vi "图像采集与保存-简单图像处理.vi"(9 "Grab":bool, 11 "Camera Name":refnum<k21>="cam0" caption="IMAQdx Session") -> ()   [LabVIEW 2022 SP3]
doc: "The Grab and Attributes Setup example VI allows the user to view the current attributes and settings, update attribute settings, acquire images continuously, and display the images in an image control."
uses:
  <vilib>/vision/driver/IMAQdx.llb/IMAQdx Acquisition Mode.ctl
  <vilib>/vision/driver/IMAQdx.llb/IMAQdx Buffer Number Mode.ctl
  <vilib>/vision/driver/NI_Vision_Acquisition_Software.lvlib
panel:
  out "Image out":T1(plugin-control)
  out "错误输出":errorcluster
  out "返回值":i32
  out "处理图片路径":path
  out "采集图片路径":path
  out "帧数":i32
  in  "采集帧间隔":i8
  in  "确定按钮":bool
  in  "Tab Control":T2(tab)
  in  "U32 Value Control":u32(slide) min=1 step=1 scale=1.0..4294967295.0
  in  "DBL Value Control":dbl(slide) min=2.2571161239684447 max=1000.0 step=1.0 scale=2.2571161239684447..1000.0
  in  "String Value Control":string
  in  "Enum Value Control":u32(ring) items=["Unicast", "Broadcast", "Multicast"]
  in  "Boolean Value Control":bool
  in  "Command Value Control":bool
  out "Tooltip":string="Gets/Sets the maximum number of outstanding events to queue."
  out "Units":string
  in  "Attribute Tree":string(tree)
  out "Frame Rate":dbl(knob) scale=0.0..100.0
  out "Image":T1(plugin-control)
  out "Buffer Number":u32
  in  "Stop":bool
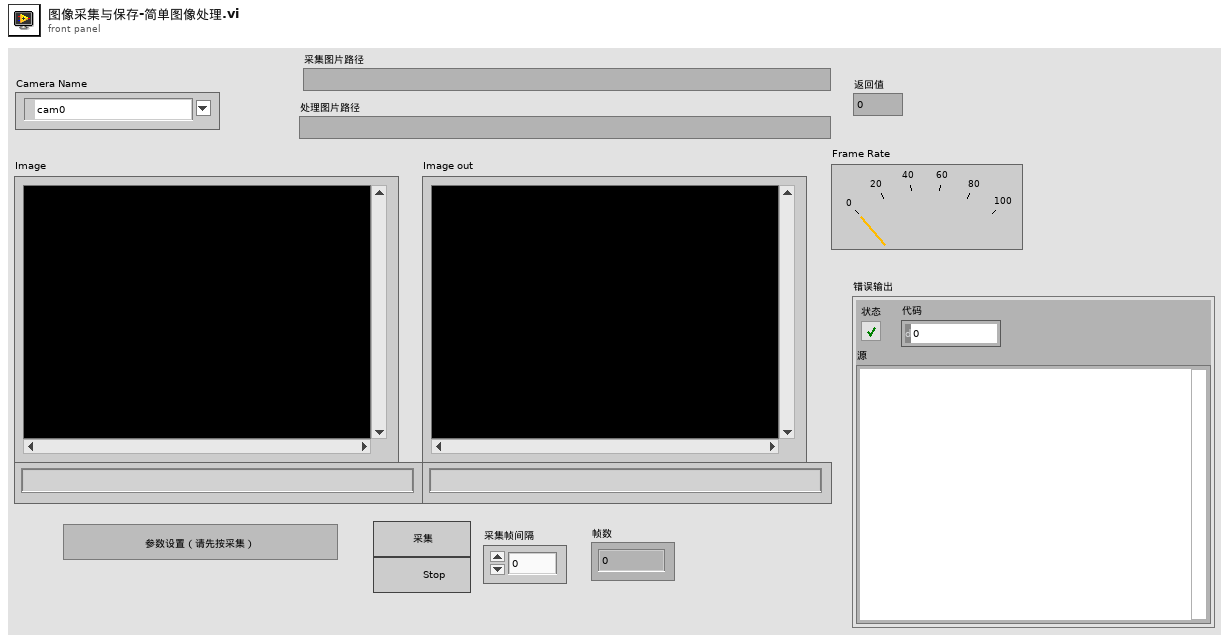
[diagram p1: front panel]
types:
  T1 = typedef "IMAQ Image.ctl" = refnum<image>
  T2 = enum32{"U32", "DBL", "String", "Enum", "Bool", "Command"}
  T3 = typedef "NI_Vision_Acquisition_Software.lvlib/IMAQdx Acquisition Mode.ctl" = enum32{"One Shot", "Continuous"}
  T4 = typedef "IMAQdx.ctl" = refnum<k21>
  T5 = cluster{"Tab Control":refnum<vi>, "U32 Value Control":refnum<vi>, "DBL Value Control":refnum<vi>, "String Value Control":refnum<vi>, "Enum Value Control":refnum<vi>, "Boolean Value Control":refnum<vi>, "Command Value Control":refnum<vi>}
  T6 = typedef "NI_Vision_Acquisition_Software.lvlib/IMAQdx Buffer Number Mode.ctl" = enum32{"Next", "Last", "Buffer Number", "Every", "Last New"}
  T7 = typedef "Image Type" = u32
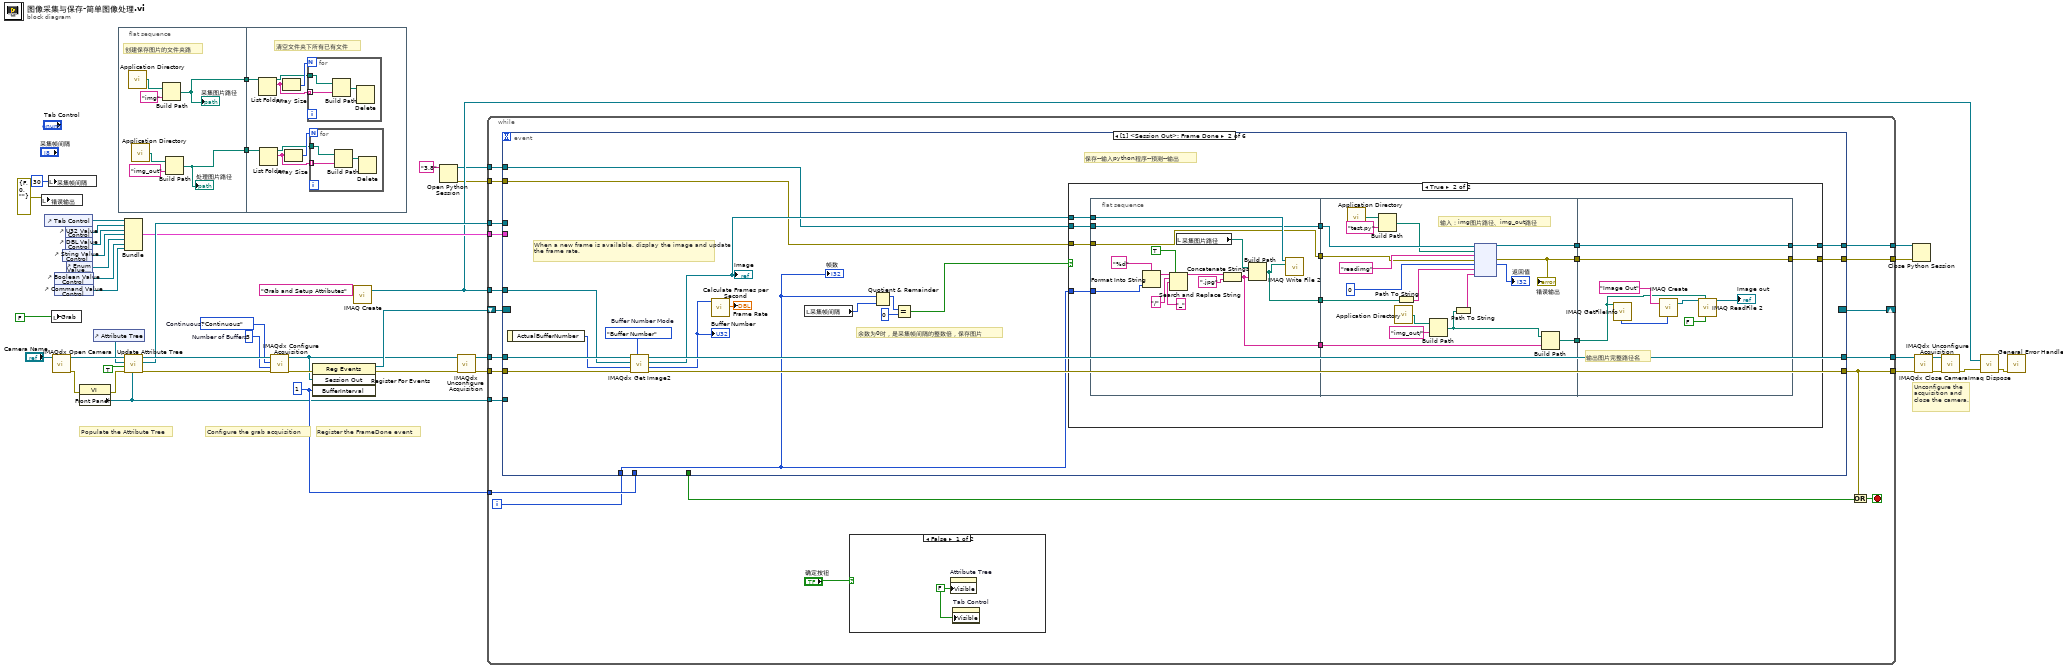
[diagram p0: block diagram]
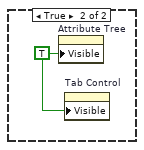
[diagram p2: hidden frame]
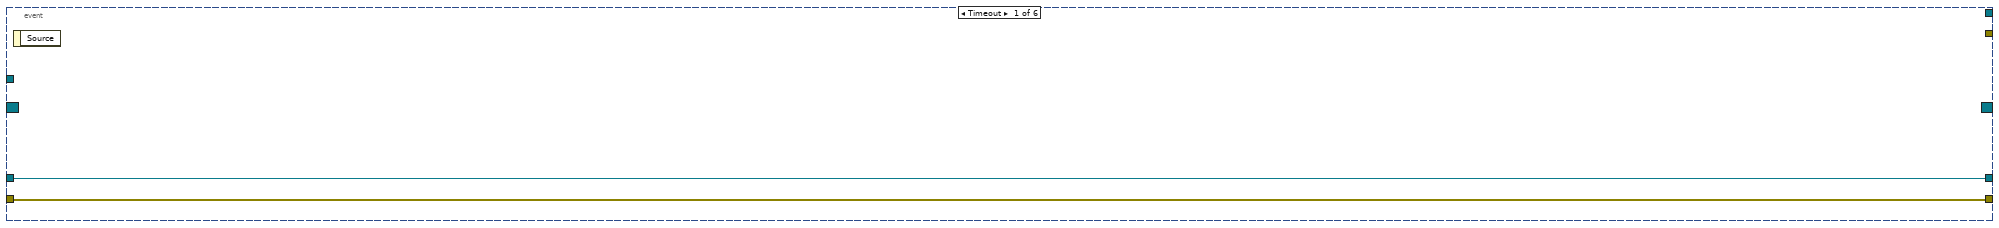
[diagram p3: hidden frame]
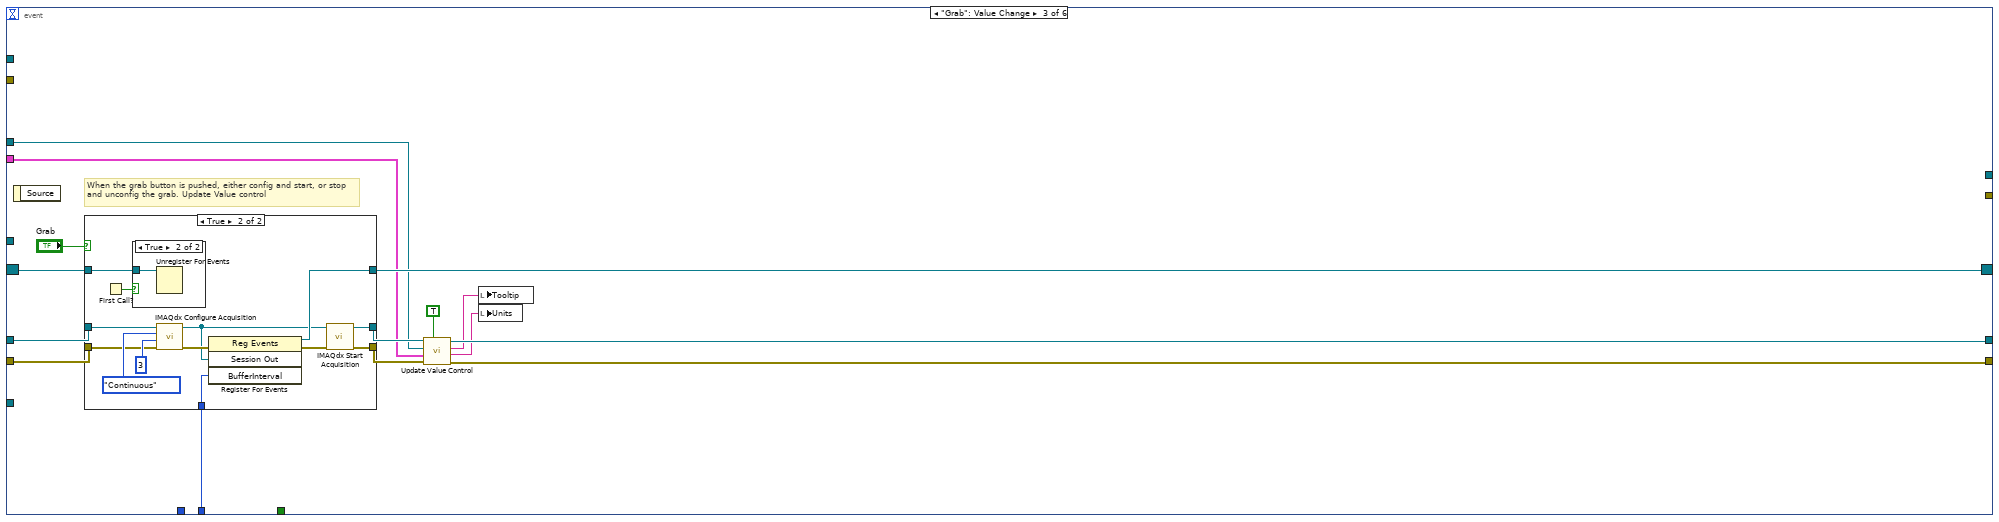
[diagram p5: hidden frame]
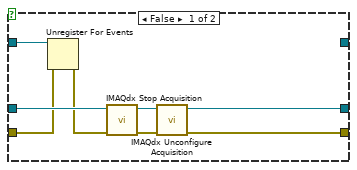
[diagram p6: hidden frame]
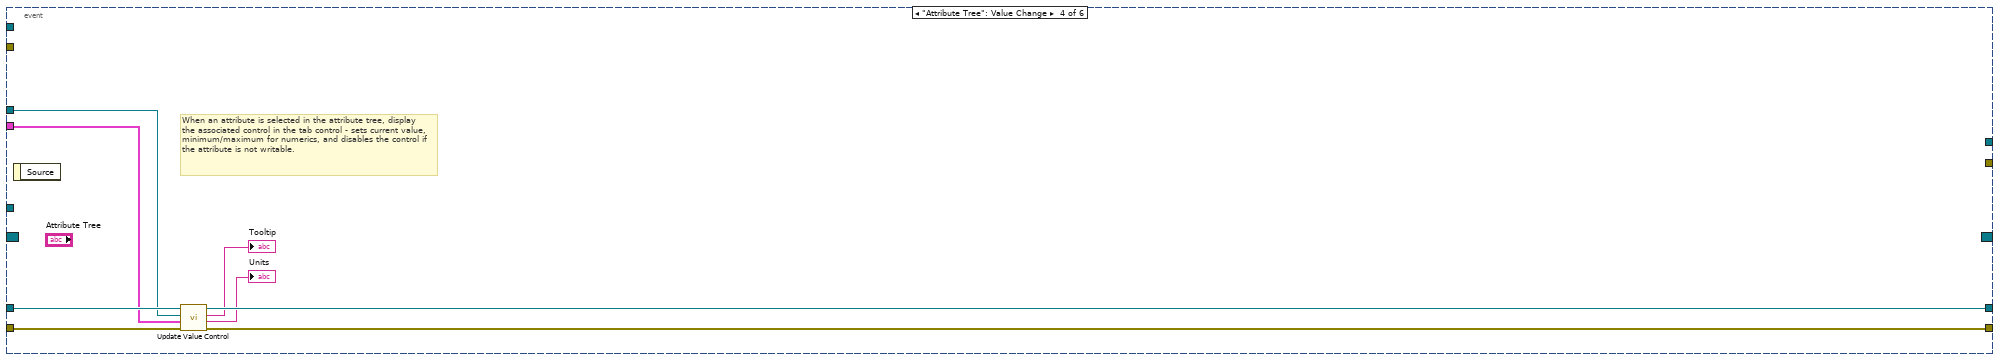
[diagram p8: hidden frame]
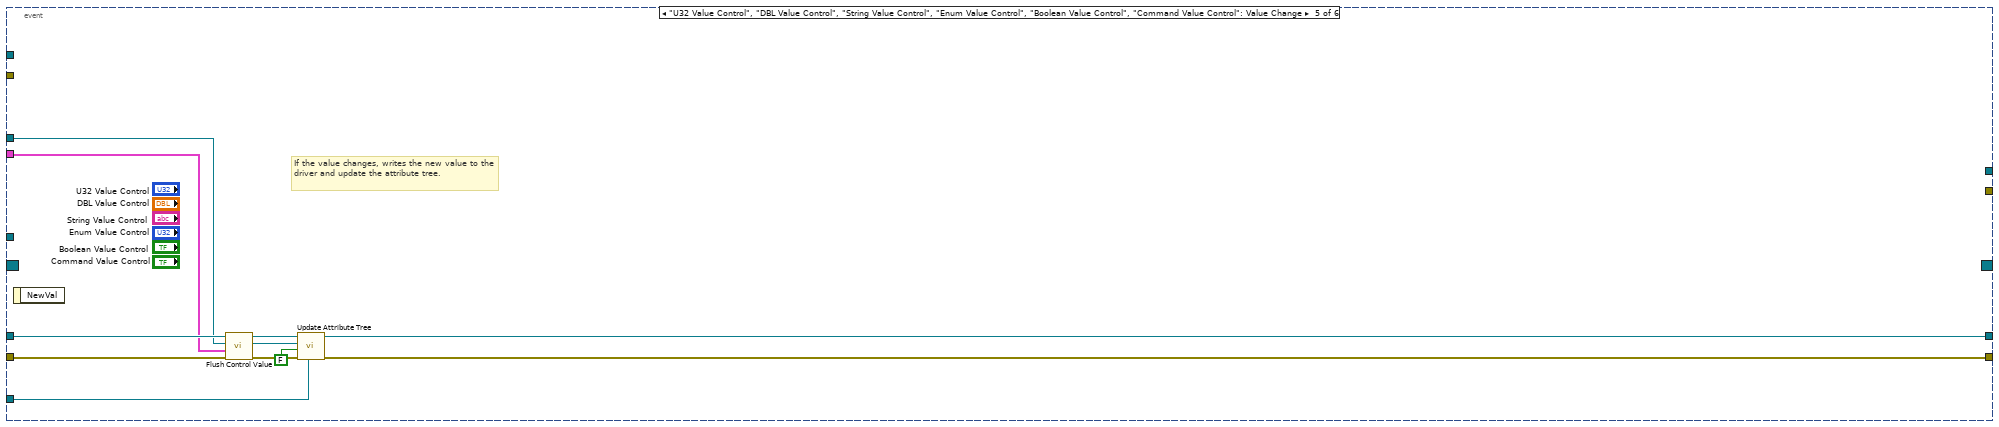
[diagram p9: hidden frame]
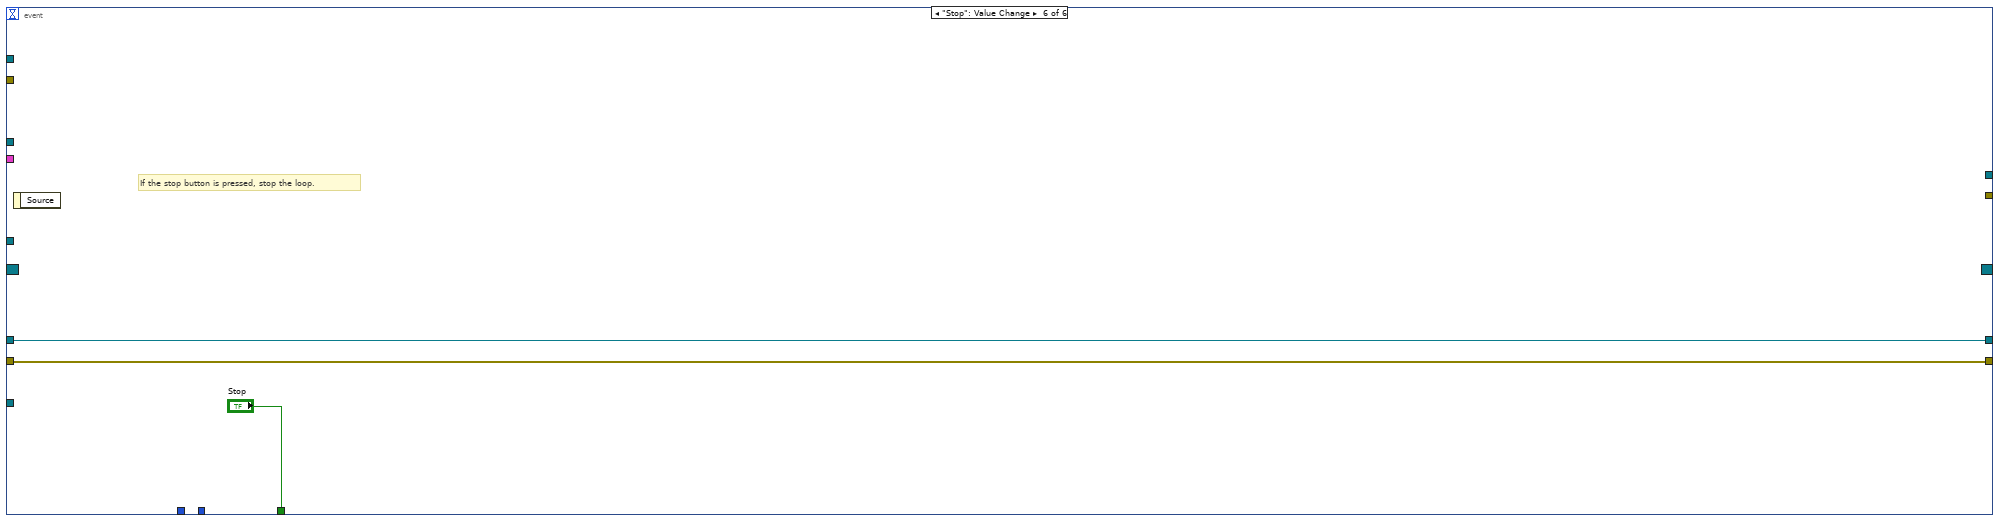
[diagram p10: hidden frame]
diagram:
  w26 = u32 1 ("BufferInterval")
  w12 = u32 3  # Number of Buffers
  w11 = IMAQdx_Acquisition_Mode."Continuous"  # Continuous?
  # "Unconfigure the acquisition and close the camera."
  # "Register the FrameDone event"
  # "Configure the grab acquisition"
  # "Populate the Attribute Tree"
  n1 = local write "错误输出"(errorcluster {"status"=FALSE, "code"=0, "source"=""} ("错误输出")) -> ()
  n2 = control-ref of="Tab Control"() -> (w16:refnum<vi>)
  n3 = local write "采集帧间隔"(i8 30 ("采集帧间隔")) -> ()
  n4 = local write "Grab"(FALSE ("Grab")) -> ()
  n5 = call <vilib>:"IMAQdx Open Camera.vi"("Session In"="Camera Name") -> ("error out"=w29:errorcluster, "Session Out"=w34:T4)  [unwired: 2 in, 7 out]
  n6 = control-ref of="Boolean Value Control"() -> (w36:refnum<vi>)
  n7 = control-ref of="Command Value Control"() -> (w35:refnum<vi>)
  n8 = control-ref of="String Value Control"() -> (w40:refnum<vi>)
  n9 = control-ref of="U32 Value Control"() -> (w39:refnum<vi>)
  n10 = control-ref of="DBL Value Control"() -> (w38:refnum<vi>)
  n11 = control-ref of="Enum Value Control"() -> (w37:refnum<vi>)
  n12 = property class="VI"(error in=w29) -> (error out=w15:errorcluster, "Front Panel"=w13:refnum<vi>)  [unwired: 1 in, 1 out]
  n13 = control-ref of="Attribute Tree"() -> (w32:refnum<vi>)
  n14 = flat-sequence {
    tunnel: [w49] -> w9
    tunnel: [w46] -> w7
    tunnel: w9 -> [w56]
    tunnel: w7 -> [w52]
    frame #0 {
      # "创建保存图片的文件夹路"
      n15 = call <vilib>:"Application Directory.vi"() -> ("Application Directory"=w51:path)
      n16 = call <vilib>:"Application Directory.vi"() -> ("Application Directory"=w48:path)
      n17 = Build Path(base path=w51, name or relative path="img" ("名称或相对路径")) -> (appended path=w49:path)
      "采集图片路径" <- w49
      n18 = Build Path(base path=w48, name or relative path="img_out" ("名称或相对路径")) -> (appended path=w46:path)
      "处理图片路径" <- w46
    }
    frame #1 {
      # "清空文件夹下所有已有文件"
      n19 = List Folder(path=w56) -> (path out=w57:path, filenames=w59:string[])  [unwired: 3 in, 2 out]
      n20 = List Folder(path=w52) -> (path out=w53:path, filenames=w55:string[])  [unwired: 3 in, 2 out]
      n21 = Array Size(array=w59) -> (size(s)=w58:i32)
      n22 = Array Size(array=w55) -> (size(s)=w54:i32)
      n23 = for {
        N: w58 -> [_]
        tunnel: w57 -> [w64]
        tunnel: w59 -> [w63] mode=indexing
        n24 = Build Path(base path=w64, name or relative path=w63) -> (appended path=w65:path)
        n25 = Delete(path (use dialog)=w65) -> ()  [unwired: 4 in, 3 out]
      }
      n26 = for {
        N: w54 -> [_]
        tunnel: w53 -> [w61]
        tunnel: w55 -> [w60] mode=indexing
        n27 = Build Path(base path=w61, name or relative path=w60) -> (appended path=w62:path)
        n28 = Delete(path (use dialog)=w62) -> ()  [unwired: 4 in, 3 out]
      }
    }
  }
  n29 = Bundle("Tab Control"=w16, "U32 Value Control"=w39, "DBL Value Control"=w38, "String Value Control"=w40, "Enum Value Control"=w37, "Boolean Value Control"=w36, "Command Value Control"=w35) -> (w21:T5)  [unwired: 1 out]
  n30 = call "Update Attribute Tree.vi"("Panel Refnum In"=w13, "error in"=w15, "Flush Tree?"=TRUE, "Tree Control In"=w32, "Camera Name In"=w34) -> ("error out"=w14:errorcluster, "Tree Control Out"=w30:refnum<vi>, "Session Out"=w33:T4)  [unwired: 4 in]
  n31 = call <vilib>:"IMAQdx Configure Acquisition.vi"("error in"=w14, "Number of Buffers"=w12, "Continuous?"=w11, "Session In"=w33) -> ("error out"=w42:errorcluster, "Session Out"=w23:T4)  [unwired: 6 out]
  n32 = register-events(error in=w42, w23, w26) -> (reference out=w41:refnum<event-registration>, error out=w25:errorcluster)  [unwired: 1 in]
  n33 = call "IMAQ Create"("Image Name"="Grab and Setup Attributes") -> ("New Image"=w18:T1)  [unwired: 3 in, 2 out]
  n34 = Open Python Session(python version="3.8" ("Python版本")) -> (session out=w5:refnum<k35>, error out=w2:errorcluster)  [unwired: 2 in]
  n35 = call <vilib>:"IMAQdx Unconfigure Acquisition.vi"("error in"=w25, "Session In"=w23) -> ("error out"=w24:errorcluster, "Session Out"=w22:T4)  [unwired: 8 out]
  n36 = while {
    tunnel: [w80] -> w28
    tunnel: w24 -> [w82]
    tunnel: w22 -> [w83]
    tunnel: [w73] -> w27
    tunnel: w18 -> [w81]
    tunnel: w30 -> [w78]
    tunnel: w13 -> [w77]
    tunnel: w26 -> [w75]
    shift-right: [w74] -> _
    shift-left: w41 -> [w79]
    tunnel: w21 -> [w72]
    tunnel: w5 -> [w69]
    tunnel: [w68] -> w4
    tunnel: [w67] -> w3
    tunnel: w2 -> [w66]
    i -> [w71]
    stop <- w84 stop-if-true
    n37 = event shown="[1] <Session Out>: Frame Done" {
      selector: w79 -> [_ _ w173 _ _ _]
      dyn-events: [_ _ w175 _ _ _] -> w74
      timeout: _ -> [_ _ _ _ _ _]
      tunnel: w83 -> [w87 w107 w177 w207 w217 w219]
      tunnel: w82 -> [w88 w106 w172 w205 w218 w220]
      tunnel: w81 -> [_ w105 _ _ _ _]
      tunnel: [w87 w104 w165 w206 w213 w219] -> w80
      tunnel: [w88 w103 w169 w204 w209 w220] -> w73
      tunnel: w78 -> [_ _ w168 w202 w211 _]
      tunnel: w77 -> [_ _ _ _ w208 _]
      tunnel: [_ _ _ _ _ "Stop"] -> w76
      tunnel: w75 -> [_ _ w174 _ _ _]
      tunnel: w72 -> [_ _ w166 w203 w212 _]
      tunnel: w71 -> [_ w95 _ _ _ _]
      tunnel: w69 -> [_ w92 _ _ _ _]
      tunnel: [_ w91 _ _ _ _] -> w68
      tunnel: [_ w90 _ _ _ _] -> w67
      tunnel: w66 -> [_ w89 _ _ _ _]
      event Timeout {
        n38 = event-data() -> ()  [unwired: 2 out]
      }
      event event #0x0 {
        w102 = IMAQdx_Buffer_Number_Mode."Buffer Number"  # Buffer Number Mode
        # "余数为0时，是采集帧间隔的整数倍，保存图片"
        # "保存--输入python程序--预测--输出"
        # "When a new frame is available, display the image and update the frame rate."
        n39 = event-data() -> ("ActualBufferNumber"=w101:u32)  [unwired: 1 out]
        n40 = call <vilib>:"IMAQdx Get Image2.vi"("Buffer Number Mode (Next)"=w102, "error in"=w106, "Buffer Number In"=w101, "Image In"=w105, "Session In"=w107) -> ("error out"=w103:errorcluster, "Buffer Number Out"=w100:u32, "Image Out"=w96:T1, "Session Out"=w104:T4)  [unwired: 3 in]
        "Image" <- w96
        "Buffer Number" <- w100
        n41 = call <vilib>:"Calculate Frames per Second.vi"("Buffer Number"=w100) -> ("Processed Frames/s"=→"Frame Rate":dbl)  [unwired: 8 in, 2 out]
        n42 = local read "采集帧间隔"() -> (w94:i8)
        n43 = Quotient & Remainder(x=w95, y=w94) -> (x-y*floor(x/y)=w93:i32)  [unwired: 1 out]
        n44 = Equal?(x=w93, y=i8 0) -> (x = y?=w97:bool)
        n45 = case shown="True" w97 {
          tunnel: w95 -> [_ w122]
          tunnel: w96 -> [_ w121]
          tunnel: w92 -> [w109 w119]
          tunnel: [w109 w117] -> w91
          tunnel: [w108 w116] -> w90
          tunnel: w89 -> [w108 w115]
          frame False {
          }
          frame True {
            n46 = flat-sequence {
              tunnel: w122 -> [w129]
              tunnel: w121 -> [w128]
              tunnel: [w126] -> w120
              tunnel: w119 -> [w126]
              tunnel: [w125] -> w118
              tunnel: w115 -> [w124]
              tunnel: [w124] -> w114
              tunnel: [w123] -> w111
              tunnel: w120 -> [w154]
              tunnel: w118 -> [w148]
              tunnel: w114 -> [w143]
              tunnel: [w145] -> w113
              tunnel: [w144] -> w112
              tunnel: w111 -> [w138]
              tunnel: [w137] -> w110
              tunnel: [w161] -> w116
              tunnel: [w162] -> w117
              tunnel: w113 -> [w162]
              tunnel: w112 -> [w161]
              tunnel: w110 -> [w156]
              frame #0 {
                n47 = Format Into String(format string="%d" ("Image Name"), w129) -> (resulting string=w130:string)  [unwired: 2 in, 1 out]
                n48 = Search and Replace String(replace all?=TRUE ("替换全部？(F)"), input string=w130, search string="/" ("搜索字符串"), replace string="_" ("替换字符串(\"\")")) -> (result string=w132:string)  [unwired: 4 in, 3 out]
                n49 = local read "采集图片路径"() -> (w127:path)
                n50 = Concatenate Strings(w132, ".jpg" ("字符串")) -> (w123:string)
                n51 = Build Path(base path=w127, name or relative path=w123) -> (appended path=w125:path)
                n52 = call-poly "IMAQ Write File 2"("File Path"=w125, "Image"=w128) -> ()  [unwired: 8 in, 2 out]
              }
              frame #1 {
                # "输入：img图片路径、img_out路径"
                n53 = call <vilib>:"Application Directory.vi"() -> ("Application Directory"=w153:path)
                n54 = Build Path(base path=w153, name or relative path="test.py" ("名称或相对路径")) -> (appended path=w151:path)
                n55 = call <vilib>:"Application Directory.vi"() -> ("Application Directory"=w142:path)
                n56 = Path To String(path=w148) -> (string=w147:string)
                n57 = Build Path(base path=w142, name or relative path="img_out/" ("名称或相对路径")) -> (appended path=w139:path)
                n58 = Path To String(path=w139) -> (string=w140:string)
                n59 = node(w154, w151, "readimg" ("函数名称"), w143, 0, w147, w140) -> (w145:refnum<k35>, w144:errorcluster, →"返回值":i32)  [unwired: 2 in, 2 out]
                "错误输出" <- w144
                n60 = Build Path(base path=w139, name or relative path=w138) -> (appended path=w137:path)
              }
              frame #2 {
                # "输出图片完整路径名"
                n61 = call "IMAQ GetFileInfo"("File Path"=w156) -> ("Image Type"=w155:T7)  [unwired: 4 in, 6 out]
                n62 = call "IMAQ Create"("Image Name"="Image Out", "Image Type"=w155) -> ("New Image"=w158:T1)  [unwired: 3 in, 1 out]
                n63 = call "IMAQ ReadFile 2"("Use File Path Image Type"=FALSE, "File Path"=w156, "Image"=w158) -> ("Image Out"=→"Image out":T1)  [unwired: 4 in, 4 out]
              }
            }
          }
        }
        "帧数" <- w95
      }
      event "Grab": Value Change {
        # "When the grab button is pushed, either config and start, or stop and unconfig the grab. Update Value control"
        n64 = event-data() -> ()  [unwired: 2 out]
        n65 = case shown="True" "Grab" {
          tunnel: w177 -> [w185 w196]
          tunnel: [w182 w198] -> w171
          tunnel: [w181 w197] -> w170
          tunnel: [_ w191] -> w175
          tunnel: w174 -> [_ w189]
          tunnel: w173 -> [w180 w187]
          tunnel: w172 -> [w178 w188]
          frame False {
            n66 = Unregister For Events(event registration refnum=w180, error in=w178) -> (error out=w179:errorcluster)
            n67 = call <vilib>:"IMAQdx Stop Acquisition.vi"("error in"=w179, "Session In"=w185) -> ("error out"=w183:errorcluster, "Session Out"=w184:T4)  [unwired: 8 out]
            n68 = call <vilib>:"IMAQdx Unconfigure Acquisition.vi"("error in"=w183, "Session In"=w184) -> ("error out"=w181:errorcluster, "Session Out"=w182:T4)  [unwired: 8 out]
          }
          frame True {
            n69 = First Call?() -> (First Call?: T/F=w186:bool)
            n70 = case shown="True" w186 {
              tunnel: w187 -> [_ w199]
              frame False {
              }
              frame True {
                n71 = Unregister For Events(event registration refnum=w199) -> ()  [unwired: 1 in, 1 out]
              }
            }
            n72 = call <vilib>:"IMAQdx Configure Acquisition.vi"("error in"=w188, "Number of Buffers"=u32 3, "Continuous?"=IMAQdx_Acquisition_Mode."Continuous", "Session In"=w196) -> ("error out"=w193:errorcluster, "Session Out"=w190:T4)  [unwired: 6 out]
            n73 = register-events(error in=w193, w190, w189) -> (reference out=w191:refnum<event-registration>, error out=w192:errorcluster)  [unwired: 1 in]
            n74 = call <vilib>:"IMAQdx Start Acquisition.vi"("error in"=w192, "Session In"=w190) -> ("error out"=w197:errorcluster, "Session Out"=w198:T4)  [unwired: 8 out]
          }
        }
        n75 = call "Update Value Control.vi"("Force update?"=TRUE, "error in (no error)"=w170, "Tab Control Ref In"=w166, "Tree Control In"=w168, "Session In"=w171) -> ("error out"=w169:errorcluster, "Units"=w163:string, "Tooltip"=w164:string, "Session Out"=w165:T4)  [unwired: 3 in]
        n76 = local write "Tooltip"(w164) -> ()
        n77 = local write "Units"(w163) -> ()
      }
      event "Attribute Tree": Value Change {
        # "When an attribute is selected in the attribute tree, display the associated control in the tab control - sets current value, minimum/maximum for numerics, and disables the control if the attribute is not writable."
        n78 = event-data() -> ()  [unwired: 2 out]
        n79 = call "Update Value Control.vi"("error in (no error)"=w205, "Tab Control Ref In"=w203, "Tree Control In"=w202, "Session In"=w207) -> ("error out"=w204:errorcluster, "Units"=→"Units":string, "Tooltip"=→"Tooltip":string, "Session Out"=w206:T4)  [unwired: 4 in]
      }
      event "U32 Value Control", "DBL Value Control", "String Value Control", "Enum Value Control", "Boolean Value Control", "Command Value Control": Value Change {
        # "If the value changes, writes the new value to the driver and update the attribute tree."
        n80 = event-data() -> ()  [unwired: 2 out]
        n81 = call "Flush Control Value.vi"("error in (no error)"=w218, "Tab Control Ref In"=w212, "Tree Control In"=w211, "Session In"=w217) -> ("error out"=w210:errorcluster, "Tree Control Out"=w215:refnum<vi>, "Session Out"=w216:T4)  [unwired: 5 in]
        n82 = call "Update Attribute Tree.vi"("Panel Refnum In"=w208, "error in"=w210, "Flush Tree?"=FALSE, "Tree Control In"=w215, "Camera Name In"=w216) -> ("error out"=w209:errorcluster, "Session Out"=w213:T4)  [unwired: 4 in, 1 out]
      }
      event "Stop": Value Change {
        # "If the stop button is pressed, stop the loop."
        n83 = event-data() -> ()  [unwired: 2 out]
      }
    }
    n84 = case shown="False" "确定按钮" {
      frame False {
        w85 = FALSE ("可见")
        n85 = property on="Attribute Tree" class="Tree (strict)"("Visible"=w85) -> ()  [unwired: 2 in, 2 out]
        n86 = property on="Tab Control" class="TabCtl (strict)"("Visible"=w85) -> ()  [unwired: 2 in, 2 out]
      }
      frame True {
        w86 = TRUE ("可见")
        n87 = property on="Attribute Tree" class="Tree (strict)"("Visible"=w86) -> ()  [unwired: 2 in, 2 out]
        n88 = property on="Tab Control" class="TabCtl (strict)"("Visible"=w86) -> ()  [unwired: 2 in, 2 out]
      }
    }
    n89 = Or(x=w73, y=w76) -> (x .or. y?=w84:bool)
  }
  n90 = Close Python Session(session in=w4, error in=w3) -> ()  [unwired: 1 out]
  n91 = call <vilib>:"IMAQdx Unconfigure Acquisition.vi"("error in"=w27, "Session In"=w28) -> ("error out"=w44:errorcluster, "Session Out"=w43:T4)  [unwired: 8 out]
  n92 = call <vilib>:"IMAQdx Close Camera.vi"("error in"=w44, "Session In"=w43) -> ("error out"=w20:errorcluster)  [unwired: 9 out]
  n93 = call "Imaq Dispose"("Image"=w18, "error in (no error)"=w20) -> ("error out"=w19:errorcluster)  [unwired: 4 in]
  n94 = call <vilib>:"General Error Handler.vi"("error in (no error)"=w19) -> ()  [unwired: 2 in, 13 out]
